vi "AlignRetroMScan.vi"(2 "Data In":i16[][](array[numeric]), 3 "Process type":u16(ring) items=["Smooth M", "Smooth with Cor", "smooth B-scan"]) -> (0 "Data out":i16[][](array[numeric]))   [LabVIEW 2022 SP3]
uses:
  <vilib>/Analysis/2dsp.llb/1D Cross Correlation (DBL).vi
  <vilib>/Analysis/NI_AALPro.lvlib
  <vilib>/Analysis/NI_AALBase.lvlib
panel:
  out "Waveform Graph":dbl[][](graph)
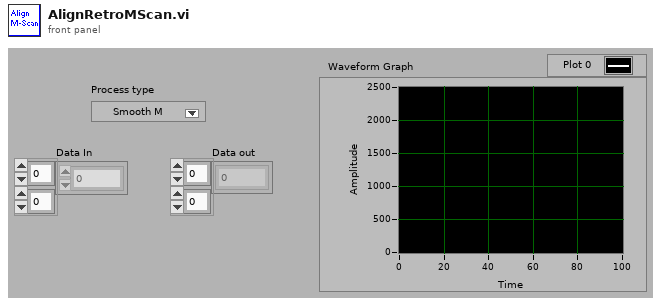
[diagram p1: front panel]
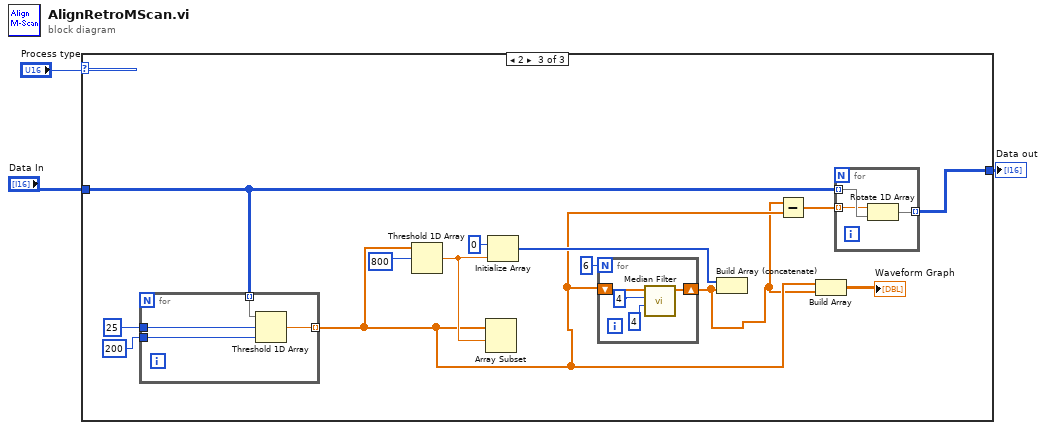
[diagram p0: block diagram]
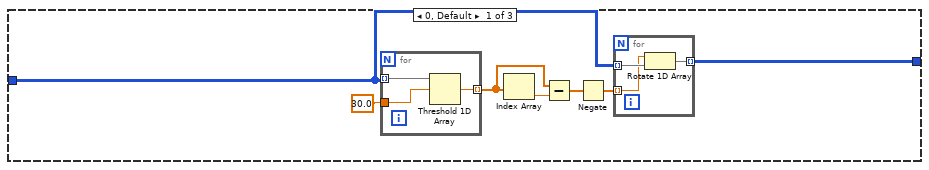
[diagram p2: hidden frame]
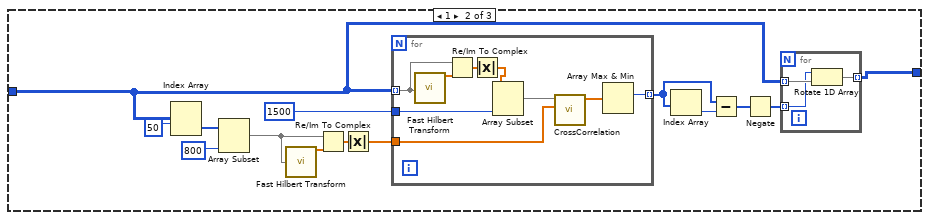
[diagram p3: hidden frame]
diagram:
  n1 = case shown="2" "Process type" {
    tunnel: [w9 w24 w47] -> w3
    tunnel: "Data In" -> [w4 w25 w48]
    frame 0, Default {
      n2 = for {
        tunnel: w4 -> [w16] mode=indexing
        tunnel: 30.0 ("threshold y") -> [w15]
        tunnel: [w14] -> w6 mode=indexing
        n3 = Threshold 1D Array(2:w15, 3:w16) -> (0:w14:dbl)  [unwired: 1 out]
      }
      n4 = Index Array(array=w6) -> (element=w5:dbl)  [unwired: 1 in]
      n5 = Subtract(x=w6, y=w5) -> (x-y=w7:dbl[])
      n6 = Negate(x=w7) -> (-x=w10:dbl[])
      n7 = for {
        tunnel: w10 -> [w12] mode=indexing
        tunnel: w4 -> [w13] mode=indexing
        tunnel: [w11] -> w9 mode=indexing
        n8 = Rotate 1D Array(1:w13, 2:w12) -> (0:w11:i16[])
      }
    }
    frame 1 {
      n9 = Index Array(array=w25, index (row)=50) -> (element=w22:i16[])  [unwired: 1 in]
      n10 = Array Subset(array=w22, length=800) -> (w18:i16[])  [unwired: 1 in]
      n11 = call <vilib>:"Fast Hilbert Transform.vi"("X"=w18) -> ("Hilbert{X}"=w20:dbl[])  [unwired: 1 out]
      n12 = Re/Im To Complex(1:w20, 2:w18) -> (0:w19:cdb[])
      n13 = Absolute Value(x=w19) -> (abs(x)=w17:dbl[])
      n14 = for {
        tunnel: w17 -> [w41]
        tunnel: w25 -> [w35] mode=indexing
        tunnel: 1500 -> [w40]
        tunnel: [w38] -> w26 mode=indexing
        n15 = call <vilib>:"Fast Hilbert Transform.vi"("X"=w35) -> ("Hilbert{X}"=w37:dbl[])  [unwired: 1 out]
        n16 = Re/Im To Complex(1:w37, 2:w35) -> (0:w36:cdb[])
        n17 = Absolute Value(x=w36) -> (abs(x)=w34:dbl[])
        n18 = Array Subset(array=w34, length=w40) -> (w42:dbl[])  [unwired: 1 in]
        n19 = call-poly <vilib>:"CrossCorrelation.vi"("Y"=w41, "X"=w42) -> ("Rxy"=w39:dbl[])  [unwired: 2 in, 7 out]
        n20 = Array Max & Min(array=w39) -> (max index (indices)=w38:i32)  [unwired: 3 out]
      }
      n21 = Index Array(array=w26) -> (element=w27:i32)  [unwired: 1 in]
      n22 = Subtract(x=w26, y=w27) -> (x-y=w28:i32[])
      n23 = Negate(x=w28) -> (-x=w29:i32[])
      n24 = for {
        tunnel: w29 -> [w32] mode=indexing
        tunnel: w25 -> [w33] mode=indexing
        tunnel: [w31] -> w24 mode=indexing
        n25 = Rotate 1D Array(1:w33, 2:w32) -> (0:w31:i16[])
      }
    }
    frame 2 {
      n26 = for {
        tunnel: 25 -> [w66]
        tunnel: [w65] -> w44 mode=indexing
        tunnel: w48 -> [w64] mode=indexing
        tunnel: 200 -> [w63]
        n27 = Threshold 1D Array(1:w63, 2:w66, 3:w64) -> (0:w65:dbl)
      }
      n28 = Threshold 1D Array(2:800, 3:w44) -> (0:w52:dbl)  [unwired: 1 out]
      n29 = Array Subset(array=w44, index=w52) -> ()  [unwired: 1 in, 1 out]
      n30 = Initialize Array(0, w52) -> (w53:i32[])
      n31 = for {
        N: 6 -> [_]
        shift-right: [w57] -> w43
        shift-left: w44 -> [w56]
        n32 = call <vilib>:"Median Filter.vi"("right rank"=4 ("polynomial order"), "left rank"=4 ("polynomial order"), "X"=w56) -> ("Filtered X"=w57:dbl[])  [unwired: 8 out]
      }
      n33 = Build Array (concatenate)(w53, w43) -> ()  [unwired: 1 out]
      n34 = Subtract(x=w43, y=w44) -> (x-y=w55:dbl[])
      n35 = Build Array(w44, w43) -> (→"Waveform Graph":dbl[][])
      n36 = for {
        tunnel: w48 -> [w62] mode=indexing
        tunnel: w55 -> [w61] mode=indexing
        tunnel: [w60] -> w47 mode=indexing
        n37 = Rotate 1D Array(1:w62, 2:w61) -> (0:w60:i16[])
      }
    }
  }
  "Data out" <- w3
